vi "Init_Spectro.vi"(8 "error in (no error)":errorcluster) -> (0 "error out":errorcluster, 2 "Wavelength_Size":i32=3648, 3 "VISA Refnum out":refnum<visa-resource-name>)   [LabVIEW 2026]
uses:
  Ocean Optics 2000 4000/Ocean Optics 2000 4000.lvlib
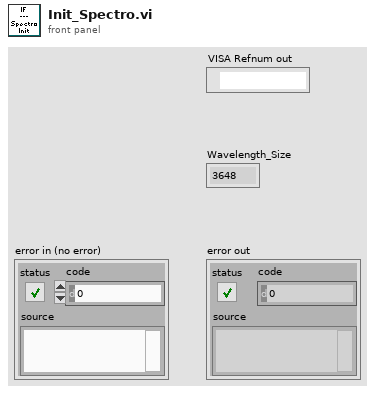
[diagram p1: front panel]
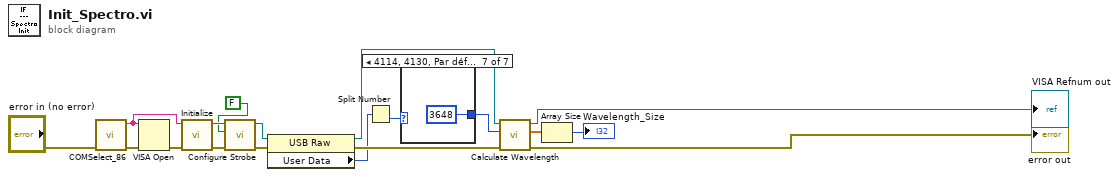
[diagram p0: block diagram]
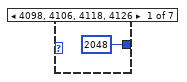
[diagram p2: hidden frame]
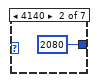
[diagram p3: hidden frame]
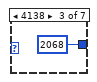
[diagram p4: hidden frame]
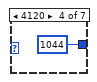
[diagram p5: hidden frame]
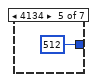
[diagram p6: hidden frame]
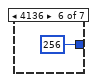
[diagram p7: hidden frame]
diagram:
  n1 = call "COMSelect_86.vi"("error in (no error)"="error in (no error)") -> ("error out"=w2:errorcluster, "COM Port Selected"=w1:string)  [unwired: 8 out]
  n2 = VISA Open(error in (no error)=w2, VISA resource name=w1) -> (error out=w16:errorcluster)  [unwired: 4 out]
  n3 = call "Initialize.vi"("error in (no error)"=w16, "VISA resource name"=w1) -> ("error out"=w15:errorcluster, "VISA resource name out"=w13:refnum<visa-resource-name>)  [unwired: 8 in]
  n4 = call "Configure Strobe.vi"("error in (no error)"=w15, "Enable Strobe (Disabled)"=FALSE, "VISA resource name"=w13) -> ("error out"=w12:errorcluster, "VISA resource name out"=w14:refnum<visa-resource-name>)  [unwired: 7 in]
  n5 = property class="USB Raw"(reference=w14, error in=w12) -> (reference out=w10:refnum<visa-resource-name>, error out=w11:errorcluster, "User Data"=w7:u32)
  n6 = Split Number(x=w7) -> (lo(x)=w8:u16)  [unwired: 1 out]
  n7 = case shown="4114, 4130, Par défaut" w8 {
    tunnel: [2048 ("Number of Pixels (3840)") 2080 ("Number of Pixels (3840)") 2068 ("Number of Pixels (3840)") 1044 ("Number of Pixels (3840)") 512 ("Number of Pixels (3840)") 256 ("Number of Pixels (3840)") 3648 ("Number of Pixels (3840)")] -> w9
    frame 4098, 4106, 4118, 4126 {
    }
    frame 4140 {
    }
    frame 4138 {
    }
    frame 4120 {
    }
    frame 4134 {
    }
    frame 4136 {
    }
    frame 4114, 4130, Default {
    }
  }
  n8 = call "Calculate Wavelength.vi"("error in (no error)"=w11, "Number of Pixels (3648)"=w9, "VISA resource name"=w10) -> ("error out"=→"error out":errorcluster, "Wavelength (nm)"=w17:dbl[], "VISA resource name out"=→"VISA Refnum out":refnum<visa-resource-name>)  [unwired: 6 in]
  n9 = Array Size(array=w17) -> (size(s)=→"Wavelength_Size":i32)
